vi "SVM Dense Cross-Validate C_SVC.vi"(6 "Nr fold":i32 caption="Nr fold (LOO)", 7 "Options":T6={"cache_size"=200.0, "eps"=0.001, "shrinking"=TRUE, "probability"=FALSE}, 8 "error in (no error)":errorcluster, 9 "Param C_SVC":T3={"C"=1.0, "weight_label"=[], "weight"=[]}, 10 "Kernel":T4, 11 "Dense problem":T1) -> (0 "error out":errorcluster, 3 "Target":dbl[](array[numeric]) caption="Target (Predicted labels)")   [LabVIEW 2014]
doc: "This function conducts cross validation. Data are separated to nr_fold folds. Under given parameters sequentially each fold is validated using the model from training the remaining. Predicted labels (of all prob's instances) in the validation process are stored in the array called target.\n\nThe default number of folds uses Leave-One-Out cross-validation (LOO)."
uses:
  LibSVM Sparse/Controls/Options Training.ctl
  LibSVM Sparse/Controls/Kernel.ctl
  LibSVM Sparse/Wrapper API/Controls/svm_kernel_type.ctl
  LibSVM Sparse/Controls/Parameters C_SVC.ctl
  Wrapper API/Controls/svmdense_problem.ctl
  Wrapper API/Controls/svmdense_node.ctl
  LibSVM Sparse/Wrapper API/Controls/svm_parameter.ctl
  LibSVM Sparse/Wrapper API/Controls/svm_type.ctl
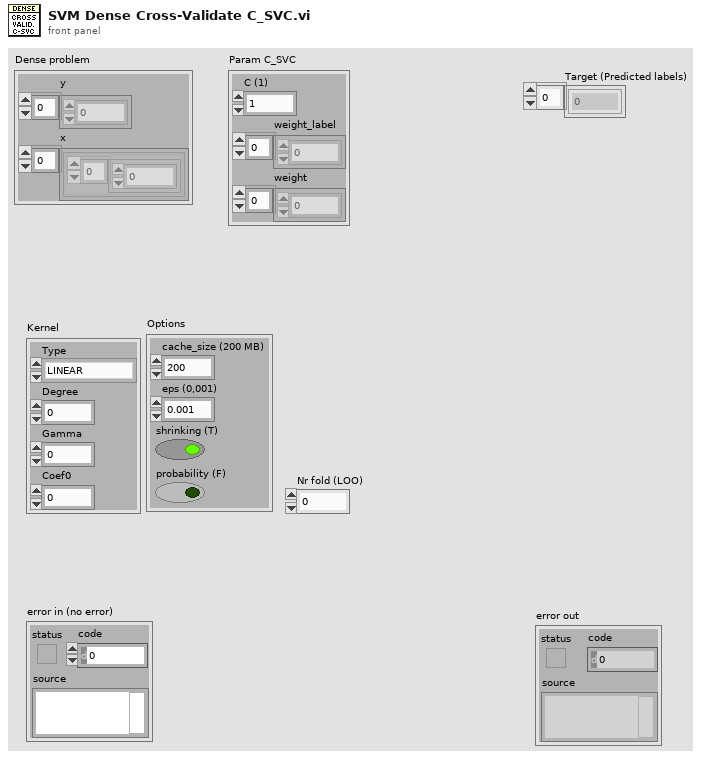
[diagram p1: front panel]
types:
  T1 = typedef "svmdense_problem.ctl" = cluster{"y":dbl[], "x":T2[]}
  T2 = typedef "svmdense_node.ctl" = cluster{"x":dbl[]}
  T3 = typedef "Parameters C_SVC.ctl" = cluster{"C":dbl, "weight_label":i32[], "weight":dbl[]}
  T4 = typedef "Kernel.ctl" = cluster{"Type":T5, "Degree":i32, "Gamma":dbl, "Coef0":dbl}
  T5 = typedef "svm_kernel_type.ctl" = enum32{"LINEAR", "POLY", "RBF", "SIGMOID", "PRECOMPUTED"}
  T6 = typedef "Options Training.ctl" = cluster{"cache_size":dbl, "eps":dbl, "shrinking":bool, "probability":bool}
  T7 = typedef "svm_type.ctl" = enum32{"C_SVC", "NU_SVC", "ONE_CLASS", "EPSILON_SVR", "NU_SVR"}
  T8 = typedef "svm_parameter.ctl" = cluster{"svm_type":T7, "kernel_type":T5, "degree":i32, "gamma":dbl, "coef0":dbl, "cache_size":dbl, "eps":dbl, "C":dbl, "weight_label":i32[], "weight":dbl[], "nu":dbl, "p":dbl, "shrinking":bool, "probability":bool}
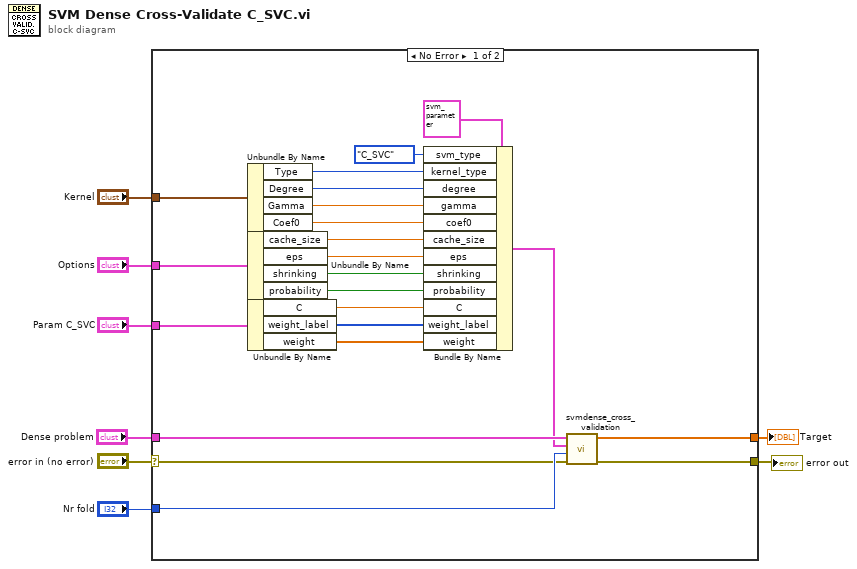
[diagram p0: block diagram]
diagram:
  n1 = case shown="No Error" "error in (no error)" {
    selector: "error in (no error)" -> [w11 w31]
    tunnel: [w9 w31] -> w8
    tunnel: "Dense problem" -> [w14 _]
    tunnel: "Kernel" -> [w29 _]
    tunnel: "Options" -> [w20 _]
    tunnel: "Param C_SVC" -> [w21 _]
    tunnel: [w10 _] -> w3
    tunnel: "Nr fold" -> [w12 _]
    frame No Error {
      n2 = Unbundle By Name(w29) -> ("Type"=w28:T5, "Degree"=w27:i32, "Gamma"=w26:dbl, "Coef0"=w25:dbl)
      n3 = Unbundle By Name(w20) -> ("cache_size"=w23:dbl, "eps"=w22:dbl, "shrinking"=w19:bool, "probability"=w18:bool)
      n4 = Unbundle By Name(w21) -> ("C"=w17:dbl, "weight_label"=w16:i32[], "weight"=w15:dbl[])
      n5 = Bundle By Name(cluster=T8 {"svm_type"=enum."C_SVC", "kernel_type"=enum."LINEAR", "degree"=0, "gamma"=0.0, "coef0"=0.0, "cache_size"=0.0, "eps"=0.0, "C"=0.0, "weight_label"=[], "weight"=[], "nu"=0.0, "p"=0.0, "shrinking"=FALSE, "probability"=FALSE} ("svm_parameter"), "svm_type"=svm_type."C_SVC", "kernel_type"=w28, "degree"=w27, "gamma"=w26, "coef0"=w25, "cache_size"=w23, "eps"=w22, "shrinking"=w19, "probability"=w18, "C"=w17, "weight_label"=w16, "weight"=w15) -> (w13:T8)
      n6 = call "svmdense_cross_validation.vi"("error in (no error)"=w11, "Nr fold"=w12, "Parameters"=w13, "Problem"=w14) -> ("error out"=w9:errorcluster, "Target"=w10:dbl[])  [unwired: 6 in]
    }
    frame Error {
    }
  }
  "error out" <- w8
  "Target" <- w3
